vi "Parameter Filter - By Channel Number.vi"(2 "Channel Number":i32, 7 "Parameters Array (in)":T1[](array[typedef])) -> (8 "Filtered Parameters Array (out)":T1[](array[typedef]))   [LabVIEW 2020] (continued)
 "Channel Speed"=100, "Label Decimal"=253, "Label Name"="Label_375", "Min Rate (mS)"=80, "Max Rate (mS)"=120, "SDI"=2, "SSM"=3, "Create SDI"=FALSE, "Create SSM"=FALSE, "Create Parity"=FALSE, "Parameter Name"="eng_rb2_lbl375_b16_28", "Start Bit"=16, "Number of Bits"=13, "Scale"="0.03125", "Offset"="0", "Signed"=TRUE, "Unit"="% Deployed", "Encoding"=enum."BNR", "Default Value"="0"}, {"Core Number"=0, "Channel Number"=23, "Channel Name"="ENG_RB2", "Channel Speed"=100, "Label Decimal"=75, "Label Name"="Label_113", "Min Rate (mS)"=160, "Max Rate (mS)"=240, "SDI"=2, "SSM"=3, "Create SDI"=FALSE, "Create SSM"=FALSE, "Create Parity"=FALSE, "Parameter Name"="eng_rb2_lbl113_b14_27", "Start Bit"=14, "Number of Bits"=14, "Scale"="0.0009765625", "Offset"="0", "Signed"=FALSE, "Unit"="IPS", "Encoding"=enum."BNR", "Default Value"="0"}, {"Core Number"=0, "Channel Number"=23, "Channel Name"="ENG_RB2", "Channel Speed"=100, "Label Decimal"=78, "Label Name"="Label_116", "Min Rate (mS)"=160, "Max Rate (mS)"=240, "SDI"=2, "SSM"=3, "Create SDI"=FALSE, "Create SSM"=FALSE, "Create Parity"=FALSE, "Parameter Name"="eng_rb2_lbl116_b14_27", "Start Bit"=14, "Number of Bits"=14, "Scale"="0.0009765625", "Offset"="0", "Signed"=FALSE, "Unit"="IPS", "Encoding"=enum."BNR", "Default Value"="0"}, {"Core Number"=0, "Channel Number"=23, "Channel Name"="ENG_RB2", "Channel Speed"=100, "Label Decimal"=79, "Label Name"="Label_117", "Min Rate (mS)"=160, "Max Rate (mS)"=240, "SDI"=2, "SSM"=3, "Create SDI"=FALSE, "Create SSM"=FALSE, "Create Parity"=FALSE, "Parameter Name"="eng_rb2_lbl117_b14_27", "Start Bit"=14, "Number of Bits"=14, "Scale"="0.0009765625", "Offset"="0", "Signed"=FALSE, "Unit"="IPS", "Encoding"=enum."BNR", "Default Value"="0"}, {"Core Number"=0, "Channel Number"=23, "Channel Name"="ENG_RB2", "Channel Speed"=100, "Label Decimal"=80, "Label Name"="Label_120", "Min Rate (mS)"=160, "Max Rate (mS)"=240, "SDI"=2, "SSM"=3, "Create SDI"=FALSE, "Create SSM"=FALSE, "Create Parity"=FALSE, "Parameter Name"="eng_rb2_lbl120_b14_27", "Start Bit"=14, "Number of Bits"=14, "Scale"="0.0009765625", "Offset"="0", "Signed"=FALSE, "Unit"="IPS", "Encoding"=enum."BNR", "Default Value"="0"}, {"Core Number"=0, "Channel Number"=23, "Channel Name"="ENG_RB2", "Channel Speed"=100, "Label Decimal"=81, "Label Name"="Label_121", "Min Rate (mS)"=160, "Max Rate (mS)"=240, "SDI"=2, "SSM"=3, "Create SDI"=FALSE, "Create SSM"=FALSE, "Create Parity"=FALSE, "Parameter Name"="eng_rb2_lbl121_b14_27", "Start Bit"=14, "Number of Bits"=14, "Scale"="0.0009765625", "Offset"="0", "Signed"=FALSE, "Unit"="IPS", "Encoding"=enum."BNR", "Default Value"="0"}, {"Core Number"=0, "Channel Number"=23, "Channel Name"="ENG_RB2", "Channel Speed"=100, "Label Decimal"=82, "Label Name"="Label_122", "Min Rate (mS)"=160, "Max Rate (mS)"=240, "SDI"=2, "SSM"=3, "Create SDI"=FALSE, "Create SSM"=FALSE, "Create Parity"=FALSE, "Parameter Name"="eng_rb2_lbl122_b14_27", "Start Bit"=14, "Number of Bits"=14, "Scale"="0.0009765625", "Offset"="0", "Signed"=FALSE, "Unit"="IPS", "Encoding"=enum."BNR", "Default Value"="0"}, {"Core Number"=0, "Channel Number"=23, "Channel Name"="ENG_RB2", "Channel Speed"=100, "Label Decimal"=83, "Label Name"="Label_123", "Min Rate (mS)"=160, "Max Rate (mS)"=240, "SDI"=2, "SSM"=3, "Create SDI"=FALSE, "Create SSM"=FALSE, "Create Parity"=FALSE, "Parameter Name"="eng_rb2_lbl123_b13_27", "Start Bit"=13, "Number of Bits"=15, "Scale"="0.0078125", "Offset"="0", "Signed"=FALSE, "Unit"="% Shaftspeed", "Encoding"=enum."BNR", "Default Value"="0"}, {"Core Number"=0, "Channel Number"=23, "Channel Name"="ENG_RB2", "Channel Speed"=100, "Label Decimal"=84, "Label Name"="Label_124", "Min Rate (mS)"=160, "Max Rate (mS)"=240, "SDI"=2, "SSM"=3, "Create SDI"=FALSE, "Create SSM"=FALSE, "Create Parity"=FALSE, "Parameter Name"="eng_rb2_lbl124_b13_27", "Start Bit"=13, "Number of Bits"=15, "Scale"="0.0078125", "Offset"="0", "Signed"=FALSE, "Unit"="% Shaftspeed", "Encoding"=enum."BNR", "Default Value"="0"}, {"Core Number"=0, "Channel Number"=23, "Channel Name"="ENG_RB2", "Channel Speed"=100, "Label Decimal"=87, "Label Name"="Label_127", "Min Rate (mS)"=160, "Max Rate (mS)"=240, "SDI"=2, "SSM"=3, "Create SDI"=FALSE, "Create SSM"=FALSE, "Create Parity"=FALSE, "Parameter Name"="eng_rb2_lbl127_b19_27", "Start Bit"=19, "Number of Bits"=9, "Scale"="1", "Offset"="0", "Signed"=FALSE, "Unit"="Deg", "Encoding"=enum."BNR", "Default Value"="0"}, {"Core Number"=0, "Channel Number"=23, "Channel Name"="ENG_RB2", "Channel Speed"=100, "Label Decimal"=93, "Label Name"="Label_135", "Min Rate (mS)"=160, "Max Rate (mS)"=240, "SDI"=2, "SSM"=3, "Create SDI"=FALSE, "Create SSM"=FALSE, "Create Parity"=FALSE, "Parameter Name"="eng_rb2_lbl135_b19_27", "Start Bit"=19, "Number of Bits"=9, "Scale"="1", "Offset"="0", "Signed"=FALSE, "Unit"="Deg", "Encoding"=enum."BNR", "Default Value"="0"}, {"Core Number"=0, "Channel Number"=23, "Channel Name"="ENG_RB2", "Channel Speed"=100, "Label Decimal"=94, "Label Name"="Label_136", "Min Rate (mS)"=160, "Max Rate (mS)"=240, "SDI"=2, "SSM"=3, "Create SDI"=FALSE, "Create SSM"=FALSE, "Create Parity"=FALSE, "Parameter Name"="eng_rb2_lbl136_b19_27", "Start Bit"=19, "Number of Bits"=9, "Scale"="1", "Offset"="0", "Signed"=FALSE, "Unit"="Deg", "Encoding"=enum."BNR", "Default Value"="0"}, {"Core Number"=0, "Channel Number"=23, "Channel Name"="ENG_RB2", "Channel Speed"=100, "Label Decimal"=95, "Label Name"="Label_137", "Min Rate (mS)"=160, "Max Rate (mS)"=240, "SDI"=2, "SSM"=3, "Create SDI"=FALSE, "Create SSM"=FALSE, "Create Parity"=FALSE, "Parameter Name"="eng_rb2_lbl137_b19_27", "Start Bit"=19, "Number of Bits"=9, "Scale"="1", "Offset"="0", "Signed"=FALSE, "Unit"="Deg", "Encoding"=enum."BNR", "Default Value"="0"}, {"Core Number"=0, "Channel Number"=23, "Channel Name"="ENG_RB2", "Channel Speed"=100, "Label Decimal"=77, "Label Name"="Label_115", "Min Rate (mS)"=160, "Max Rate (mS)"=240, "SDI"=2, "SSM"=3, "Create SDI"=FALSE, "Create SSM"=FALSE, "Create Parity"=FALSE, "Parameter Name"="eng_rb2_lbl115_b17_28", "Start Bit"=17, "Number of Bits"=12, "Scale"="0.25", "Offset"="0", "Signed"=TRUE, "Unit"="Degrees C", "Encoding"=enum."BNR", "Default Value"="0"}, {"Core Number"=0, "Channel Number"=23, "Channel Name"="ENG_RB2", "Channel Speed"=100, "Label Decimal"=164, "Label Name"="Label_244", "Min Rate (mS)"=160, "Max Rate (mS)"=240, "SDI"=2, "SSM"=3, "Create SDI"=FALSE, "Create SSM"=FALSE, "Create Parity"=FALSE, "Parameter Name"="eng_rb2_lbl244_b12_27", "Start Bit"=12, "Number of Bits"=16, "Scale"="0.25", "Offset"="0", "Signed"=FALSE, "Unit"="pph", "Encoding"=enum."BNR", "Default Value"="0"}, {"Core Number"=0, "Channel Number"=23, "Channel Name"="ENG_RB2", "Channel Speed"=100, "Label Decimal"=206, "Label Name"="Label_316", "Min Rate (mS)"=160, "Max Rate (mS)"=240, "SDI"=2, "SSM"=3, "Create SDI"=FALSE, "Create SSM"=FALSE, "Create Parity"=FALSE, "Parameter Name"="eng_rb2_lbl316_b16_28", "Start Bit"=16, "Number of Bits"=13, "Scale"="0.25", "Offset"="0", "Signed"=TRUE, "Unit"="Degrees C", "Encoding"=enum."BNR", "Default Value"="0"}, {"Core Number"=0, "Channel Number"=23, "Channel Name"="ENG_RB2", "Channel Speed"=100, "Label Decimal"=207, "Label Name"="Label_317", "Min Rate (mS)"=160, "Max Rate (mS)"=240, "SDI"=2, "SSM"=3, "Create SDI"=FALSE, "Create SSM"=FALSE, "Create Parity"=FALSE, "Parameter Name"="eng_rb2_lbl317_b14_27", "Start Bit"=14, "Number of Bits"=14, "Scale"="0.0625", "Offset"="0", "Signed"=FALSE, "Unit"="Psid", "Encoding"=enum."BNR", "Default Value"="0"}, {"Core Number"=0, "Channel Number"=23, "Channel Name"="ENG_RB2", "Channel Speed"=100, "Label Decimal"=162, "Label Name"="Label_242", "Min Rate (mS)"=800, "Max Rate (mS)"=1200, "SDI"=2, "SSM"=3, "Create SDI"=FALSE, "Create SSM"=FALSE, "Create Parity"=FALSE, "Parameter Name"="eng_rb2_lbl242_b18_27", "Start Bit"=18, "Number of Bits"=10, "Scale"="0.0078125", "Offset"="0", "Signed"=FALSE, "Unit"="lbm/s", "Encoding"=enum."BNR", "Default Value"="0"}, {"Core Number"=0, "Channel Number"=23, "Channel Name"="ENG_RB2", "Channel Speed"=100, "Label Decimal"=192, "Label Name"="Label_300", "Min Rate (mS)"=800, "Max Rate (mS)"=1200, "SDI"=2, "SSM"=3, "Create SDI"=FALSE, "Create SSM"=FALSE, "Create Parity"=FALSE, "Parameter Name"="eng_rb2_lbl300_b17_28", "Start Bit"=17, "Number of Bits"=12, "Scale"="0.125", "Offset"="0", "Signed"=TRUE, "Unit"="Deg C", "Encoding"=enum."BNR", "Default Value"="0"}, {"Core Number"=0, "Channel Number"=23, "Channel Name"="ENG_RB2", "Channel Speed"=100, "Label Decimal"=148, "Label Name"="Label_224", "Min Rate (mS)"=800, "Max Rate (mS)"=1200, "SDI"=2, "SSM"=3, "Create SDI"=FALSE, "Create SSM"=FALSE, "Create Parity"=FALSE, "Parameter Name"="eng_rb2_lbl224_b12_27", "Start Bit"=12, "Number of Bits"=16, "Scale"="1", "Offset"="0", "Signed"=FALSE, "Unit"="N/A", "Encoding"=enum."BNR", "Default Value"="0"}, {"Core Number"=0, "Channel Number"=23, "Channel Name"="ENG_RB2", "Channel Speed"=100, "Label Decimal"=149, "Label Name"="Label_225", "Min Rate (mS)"=800, "Max Rate (mS)"=1200, "SDI"=2, "SSM"=3, "Create SDI"=FALSE, "Create SSM"=FALSE, "Create Parity"=FALSE, "Parameter Name"="eng_rb2_lbl225_b12_27", "Start Bit"=12, "Number of Bits"=16, "Scale"="1", "Offset"="0", "Signed"=FALSE, "Unit"="N/A", "Encoding"=enum."BNR", "Default Value"="0"}, {"Core Number"=0, "Channel Number"=23, "Channel Name"="ENG_RB2", "Channel Speed"=100, "Label Decimal"=133, "Label Name"="Label_205", "Min Rate (mS)"=800, "Max Rate (mS)"=1200, "SDI"=2, "SSM"=3, "Create SDI"=FALSE, "Create SSM"=FALSE, "Create Parity"=FALSE, "Parameter Name"="eng_rb2_lbl205_b12_27", "Start Bit"=12, "Number of Bits"=16, "Scale"="0.0000625", "Offset"="0", "Signed"=FALSE, "Unit"="Mach", "Encoding"=enum."BNR", "Default Value"="0"}, {"Core Number"=0, "Channel Number"=23, "Channel Name"="ENG_RB2", "Channel Speed"=100, "Label Decimal"=168, "Label Name"="Label_250", "Min Rate (mS)"=800, "Max Rate (mS)"=1200, "SDI"=2, "SSM"=3, "Create SDI"=FALSE, "Create SSM"=FALSE, "Create Parity"=FALSE, "Parameter Name"="eng_rb2_lbl250_b15_27", "Start Bit"=15, "Number of Bits"=13, "Scale"="0.00048828125", "Offset"="0", "Signed"=FALSE, "Unit"="Pressure ratio", "Encoding"=enum."BNR", "Default Value"="0"}, {"Core Number"=0, "Channel Number"=23, "Channel Name"="ENG_RB2", "Channel Speed"=100, "Label Decimal"=171, "Label Name"="Label_253", "Min Rate (mS)"=800, "Max Rate (mS)"=1200, "SDI"=2, "SSM"=3, "Create SDI"=FALSE, "Create SSM"=FALSE, "Create Parity"=FALSE, "Parameter Name"="eng_rb2_lbl253_b15_27", "Start Bit"=15, "Number of Bits"=13, "Scale"="0.00048828125", "Offset"="0", "Signed"=FALSE, "Unit"="Pressure ratio", "Encoding"=enum."BNR", "Default Value"="0"}, {"Core Number"=0, "Channel Number"=23, "Channel Name"="ENG_RB2", "Channel Speed"=100, "Label Decimal"=173, "Label Name"="Label_255", "Min Rate (mS)"=800, "Max Rate (mS)"=1200, "SDI"=2, "SSM"=3, "Create SDI"=FALSE, "Create SSM"=FALSE, "Create Parity"=FALSE, "Parameter Name"="eng_rb2_lbl255_b15_27", "Start Bit"=15, "Number of Bits"=13, "Scale"="0.00048828125", "Offset"="0", "Signed"=FALSE, "Unit"="Pressure ratio", "Encoding"=enum."BNR", "Default Value"="0"}, {"Core Number"=0, "Channel Number"=23, "Channel Name"="ENG_RB2", "Channel Speed"=100, "Label Decimal"=223, "Label Name"="Label_337", "Min Rate (mS)"=800, "Max Rate (mS)"=1200, "SDI"=2, "SSM"=3, "Create SDI"=FALSE, "Create SSM"=FALSE, "Create Parity"=FALSE, "Parameter Name"="eng_rb2_lbl337_b15_27", "Start Bit"=15, "Number of Bits"=13, "Scale"="0.00048828125", "Offset"="0", "Signed"=FALSE, "Unit"="Pressure ratio", "Encoding"=enum."BNR", "Default Value"="0"}, {"Core Number"=0, "Channel Number"=23, "Channel Name"="ENG_RB2", "Channel Speed"=100, "Label Decimal"=134, "Label Name"="Label_206", "Min Rate (mS)"=800, "Max Rate (mS)"=1200, "SDI"=2, "SSM"=3, "Create SDI"=FALSE, "Create SSM"=FALSE, "Create Parity"=FALSE, "Parameter Name"="eng_rb2_lbl206_b14_27", "Start Bit"=14, "Number of Bits"=14, "Scale"="0.0009765625", "Offset"="0", "Signed"=FALSE, "Unit"="IPS", "Encoding"=enum."BNR", "Default Value"="0"}, {"Core Number"=0, "Channel Number"=23, "Channel Name"="ENG_RB2", "Channel Speed"=100, "Label Decimal"=138, "Label Name"="Label_212", "Min Rate (mS)"=800, "Max Rate (mS)"=1200, "SDI"=2, "SSM"=3, "Create SDI"=FALSE, "Create SSM"=FALSE, "Create Parity"=FALSE, "Parameter Name"="eng_rb2_lbl212_b14_27", "Start Bit"=14, "Number of Bits"=14, "Scale"="0.0009765625", "Offset"="0", "Signed"=FALSE, "Unit"="IPS", "Encoding"=enum."BNR", "Default Value"="0"}, {"Core Number"=0, "Channel Number"=23, "Channel Name"="ENG_RB2", "Channel Speed"=100, "Label Decimal"=65, "Label Name"="Label_101", "Min Rate (mS)"=800, "Max Rate (mS)"=1200, "SDI"=2, "SSM"=3, "Create SDI"=FALSE, "Create SSM"=FALSE, "Create Parity"=FALSE, "Parameter Name"="eng_rb2_lbl101_b12_27", "Start Bit"=12, "Number of Bits"=16, "Scale"="1", "Offset"="0", "Signed"=FALSE, "Unit"="N/A", "Encoding"=enum."BNR", "Default Value"="0"}, {"Core Number"=0, "Channel Number"=23, "Channel Name"="ENG_RB2", "Channel Speed"=100, "Label Decimal"=67, "Label Name"="Label_103", "Min Rate (mS)"=800, "Max Rate (mS)"=1200, "SDI"=2, "SSM"=3, "Create SDI"=FALSE, "Create SSM"=FALSE, "Create Parity"=FALSE, "Parameter Name"="eng_rb2_lbl103_b12_27", "Start Bit"=12, "Number of Bits"=16, "Scale"="1", "Offset"="0", "Signed"=FALSE, "Unit"="N/A", "Encoding"=enum."BNR", "Default Value"="0"}, {"Core Number"=0, "Channel Number"=23, "Channel Name"="ENG_RB2", "Channel Speed"=100, "Label Decimal"=159, "Label Name"="Label_237", "Min Rate (mS)"=800, "Max Rate (mS)"=1200, "SDI"=2, "SSM"=3, "Create SDI"=FALSE, "Create SSM"=FALSE, "Create Parity"=FALSE, "Parameter Name"="eng_rb2_lbl237_b12_27", "Start Bit"=12, "Number of Bits"=16, "Scale"="1", "Offset"="0", "Signed"=FALSE, "Unit"="N/A", "Encoding"=enum."BNR", "Default Value"="0"}, {"Core Number"=0, "Channel Number"=23, "Channel Name"="ENG_RB2", "Channel Speed"=100, "Label Decimal"=214, "Label Name"="Label_326", "Min Rate (mS)"=800, "Max Rate (mS)"=1200, "SDI"=2, "SSM"=3, "Create SDI"=FALSE, "Create SSM"=FALSE, "Create Parity"=FALSE, "Parameter Name"="eng_rb2_lbl326_b12_27", "Start Bit"=12, "Number of Bits"=16, "Scale"="1", "Offset"="0", "Signed"=FALSE, "Unit"="N/A", "Encoding"=enum."BNR", "Default Value"="0"}, {"Core Number"=0, "Channel Number"=23, "Channel Name"="ENG_RB2", "Channel Speed"=100, "Label Decimal"=152, "Label Name"="Label_230", "Min Rate (mS)"=800, "Max Rate (mS)"=1200, "SDI"=2, "SSM"=3, "Create SDI"=FALSE, "Create SSM"=FALSE, "Create Parity"=FALSE, "Parameter Name"="eng_rb2_lbl230_b12_27", "Start Bit"=12, "Number of Bits"=16, "Scale"="1", "Offset"="0", "Signed"=FALSE, "Unit"="N/A", "Encoding"=enum."BNR", "Default Value"="0"}, {"Core Number"=0, "Channel Number"=23, "Channel Name"="ENG_RB2", "Channel Speed"=100, "Label Decimal"=215, "Label Name"="Label_327", "Min Rate (mS)"=800, "Max Rate (mS)"=1200, "SDI"=2, "SSM"=3, "Create SDI"=FALSE, "Create SSM"=FALSE, "Create Parity"=FALSE, "Parameter Name"="eng_rb2_lbl327_b12_27", "Start Bit"=12, "Number of Bits"=16, "Scale"="1", "Offset"="0", "Signed"=FALSE, "Unit"="N/A", "Encoding"=enum."BNR", "Default Value"="0"}, {"Core Number"=0, "Channel Number"=23, "Channel Name"="ENG_RB2", "Channel Speed"=100, "Label Decimal"=154, "Label Name"="Label_232", "Min Rate (mS)"=800, "Max Rate (mS)"=1200, "SDI"=2, "SSM"=3, "Create SDI"=FALSE, "Create SSM"=FALSE, "Create Parity"=FALSE, "Parameter Name"="eng_rb2_lbl232_b12_27", "Start Bit"=12, "Number of Bits"=16, "Scale"="1", "Offset"="0", "Signed"=FALSE, "Unit"="N/A", "Encoding"=enum."BNR", "Default Value"="0"}, {"Core Number"=0, "Channel Number"=23, "Channel Name"="ENG_RB2", "Channel Speed"=100, "Label Decimal"=106, "Label Name"="Label_152", "Min Rate (mS)"=800, "Max Rate (mS)"=1200, "SDI"=2, "SSM"=3, "Create SDI"=FALSE, "Create SSM"=FALSE, "Create Parity"=FALSE, "Parameter Name"="eng_rb2_lbl152_b12_27", "Start Bit"=12, "Number of Bits"=16, "Scale"="1", "Offset"="0", "Signed"=FALSE, "Unit"="N/A", "Encoding"=enum."BNR", "Default Value"="0"}, {"Core Number"=0, "Channel Number"=23, "Channel Name"="ENG_RB2", "Channel Speed"=100, "Label Decimal"=156, "Label Name"="Label_234", "Min Rate (mS)"=800, "Max Rate (mS)"=1200, "SDI"=2, "SSM"=3, "Create SDI"=FALSE, "Create SSM"=FALSE, "Create Parity"=FALSE, "Parameter Name"="eng_rb2_lbl234_b12_27", "Start Bit"=12, "Number of Bits"=16, "Scale"="1", "Offset"="0", "Signed"=FALSE, "Unit"="N/A", "Encoding"=enum."BNR", "Default Value"="0"}, {"Core Number"=0, "Channel Number"=23, "Channel Name"="ENG_RB2", "Channel Speed"=100, "Label Decimal"=135, "Label Name"="Label_207", "Min Rate (mS)"=800, "Max Rate (mS)"=1200, "SDI"=2, "SSM"=3, "Create SDI"=FALSE, "Create SSM"=FALSE, "Create Parity"=FALSE, "Parameter Name"="eng_rb2_lbl207_b12_27", "Start Bit"=12, "Number of Bits"=16, "Scale"="1", "Offset"="0", "Signed"=FALSE, "Unit"="N/A", "Encoding"=enum."BNR", "Default Value"="0"}, {"Core Number"=0, "Channel Number"=23, "Channel Name"="ENG_RB2", "Channel Speed"=100, "Label Decimal"=157, "Label Name"="Label_235", "Min Rate (mS)"=800, "Max Rate (mS)"=1200, "SDI"=2, "SSM"=3, "Create SDI"=FALSE, "Create SSM"=FALSE, "Create Parity"=FALSE, "Parameter Name"="eng_rb2_lbl235_b14_28", "Start Bit"=14, "Number of Bits"=15, "Scale"="0.0067138671875", "Offset"="0", "Signed"=TRUE, "Unit"="Psia", "Encoding"=enum."BNR", "Default Value"="0"}, {"Core Number"=0, "Channel Number"=23, "Channel Name"="ENG_RB2", "Channel Speed"=100, "Label Decimal"=43, "Label Name"="Label_53", "Min Rate (mS)"=800, "Max Rate (mS)"=1200, "SDI"=2, "SSM"=3, "Create SDI"=FALSE, "Create SSM"=FALSE, "Create Parity"=FALSE, "Parameter Name"="eng_rb2_lbl53_b14_27", "Start Bit"=14, "Number of Bits"=14, "Scale"="0.001953125", "Offset"="0", "Signed"=FALSE, "Unit"="Psia", "Encoding"=enum."BNR", "Default Value"="0"}, {"Core Number"=0, "Channel Number"=23, "Channel Name"="ENG_RB2", "Channel Speed"=100, "Label Decimal"=76, "Label Name"="Label_114", "Min Rate (mS)"=800, "Max Rate (mS)"=1200, "SDI"=2, "SSM"=3, "Create SDI"=FALSE, "Create SSM"=FALSE, "Create Parity"=FALSE, "Parameter Name"="eng_rb2_lbl114_b14_27", "Start Bit"=14, "Number of Bits"=14, "Scale"="0.001953125", "Offset"="0", "Signed"=FALSE, "Unit"="Psia", "Encoding"=enum."BNR", "Default Value"="0"}, {"Core Number"=0, "Channel Number"=23, "Channel Name"="ENG_RB2", "Channel Speed"=100, "Label Decimal"=131, "Label Name"="Label_203", "Min Rate (mS)"=800, "Max Rate (mS)"=1200, "SDI"=2, "SSM"=3, "Create SDI"=FALSE, "Create SSM"=FALSE, "Create Parity"=FALSE, "Parameter Name"="eng_rb2_lbl203_b13_28", "Start Bit"=13, "Number of Bits"=16, "Scale"="2", "Offset"="0", "Signed"=TRUE, "Unit"="Feet", "Encoding"=enum."BNR", "Default Value"="0"}, {"Core Number"=0, "Channel Number"=23, "Channel Name"="ENG_RB2", "Channel Speed"=100, "Label Decimal"=153, "Label Name"="Label_231", "Min Rate (mS)"=800, "Max Rate (mS)"=1200, "SDI"=2, "SSM"=3, "Create SDI"=FALSE, "Create SSM"=FALSE, "Create Parity"=FALSE, "Parameter Name"="eng_rb2_lbl231_b17_28", "Start Bit"=17, "Number of Bits"=12, "Scale"="0.125", "Offset"="0", "Signed"=TRUE, "Unit"="Degrees C", "Encoding"=enum."BNR", "Default Value"="0"}, {"Core Number"=0, "Channel Number"=23, "Channel Name"="ENG_RB2", "Channel Speed"=100, "Label Decimal"=195, "Label Name"="Label_303", "Min Rate (mS)"=800, "Max Rate (mS)"=1200, "SDI"=2, "SSM"=3, "Create SDI"=FALSE, "Create SSM"=FALSE, "Create Parity"=FALSE, "Parameter Name"="eng_rb2_lbl303_b15_27", "Start Bit"=15, "Number of Bits"=13, "Scale"="0.00390625", "Offset"="0", "Signed"=FALSE, "Unit"="Psia", "Encoding"=enum."BNR", "Default Value"="0"}, {"Core Number"=0, "Channel Number"=23, "Channel Name"="ENG_RB2", "Channel Speed"=100, "Label Decimal"=24, "Label Name"="Label_30", "Min Rate (mS)"=800, "Max Rate (mS)"=1200, "SDI"=2, "SSM"=3, "Create SDI"=FALSE, "Create SSM"=FALSE, "Create Parity"=FALSE, "Parameter Name"="eng_rb2_lbl30_b14_27", "Start Bit"=14, "Number of Bits"=14, "Scale"="0.03125", "Offset"="0", "Signed"=FALSE, "Unit"="Psid", "Encoding"=enum."BNR", "Default Value"="0"}, {"Core Number"=0, "Channel Number"=23, "Channel Name"="ENG_RB2", "Channel Speed"=100, "Label Decimal"=40, "Label Name"="Label_50", "Min Rate (mS)"=800, "Max Rate (mS)"=1200, "SDI"=2, "SSM"=3, "Create SDI"=FALSE, "Create SSM"=FALSE, "Create Parity"=FALSE, "Parameter Name"="eng_rb2_lbl50_b14_27", "Start Bit"=14, "Number of Bits"=14, "Scale"="0.015625", "Offset"="0", "Signed"=FALSE, "Unit"="% Shaftspeed", "Encoding"=enum."BNR", "Default Value"="0"}, {"Core Number"=0, "Channel Number"=23, "Channel Name"="ENG_RB2", "Channel Speed"=100, "Label Decimal"=41, "Label Name"="Label_51", "Min Rate (mS)"=800, "Max Rate (mS)"=1200, "SDI"=2, "SSM"=3, "Create SDI"=FALSE, "Create SSM"=FALSE, "Create Parity"=FALSE, "Parameter Name"="eng_rb2_lbl51_b14_27", "Start Bit"=14, "Number of Bits"=14, "Scale"="0.015625", "Offset"="0", "Signed"=FALSE, "Unit"="% Shaftspeed", "Encoding"=enum."BNR", "Default Value"="0"}, {"Core Number"=0, "Channel Number"=23, "Channel Name"="ENG_RB2", "Channel Speed"=100, "Label Decimal"=85, "Label Name"="Label_125", "Min Rate (mS)"=800, "Max Rate (mS)"=1200, "SDI"=2, "SSM"=3, "Create SDI"=FALSE, "Create SSM"=FALSE, "Create Parity"=FALSE, "Parameter Name"="eng_rb2_lbl125_b16_28", "Start Bit"=16, "Number of Bits"=13, "Scale"="0.125", "Offset"="0", "Signed"=TRUE, "Unit"="Degrees C", "Encoding"=enum."BNR", "Default Value"="0"}, {"Core Number"=0, "Channel Number"=23, "Channel Name"="ENG_RB2", "Channel Speed"=100, "Label Decimal"=86, "Label Name"="Label_126", "Min Rate (mS)"=800, "Max Rate (mS)"=1200, "SDI"=2, "SSM"=3, "Create SDI"=FALSE, "Create SSM"=FALSE, "Create Parity"=FALSE, "Parameter Name"="eng_rb2_lbl126_b16_28", "Start Bit"=16, "Number of Bits"=13, "Scale"="0.125", "Offset"="0", "Signed"=TRUE, "Unit"="Degrees C", "Encoding"=enum."BNR", "Default Value"="0"}, {"Core Number"=0, "Channel Number"=23, "Channel Name"="ENG_RB2", "Channel Speed"=100, "Label Decimal"=96, "Label Name"="Label_140", "Min Rate (mS)"=800, "Max Rate (mS)"=1200, "SDI"=2, "SSM"=3, "Create SDI"=FALSE, "Create SSM"=FALSE, "Create Parity"=FALSE, "Parameter Name"="eng_rb2_lbl140_b15_28", "Start Bit"=15, "Number of Bits"=14, "Scale"="0.5", "Offset"="0", "Signed"=TRUE, "Unit"="Degrees C", "Encoding"=enum."BNR", "Default Value"="0"}, {"Core Number"=0, "Channel Number"=23, "Channel Name"="ENG_RB2", "Channel Speed"=100, "Label Decimal"=116, "Label Name"="Label_164", "Min Rate (mS)"=800, "Max Rate (mS)"=1200, "SDI"=2, "SSM"=3, "Create SDI"=FALSE, "Create SSM"=FALSE, "Create Parity"=FALSE, "Parameter Name"="eng_rb2_lbl164_b14_27", "Start Bit"=14, "Number of Bits"=14, "Scale"="0.03125", "Offset"="0", "Signed"=FALSE, "Unit"="Psid", "Encoding"=enum."BNR", "Default Value"="0"}, {"Core Number"=0, "Channel Number"=23, "Channel Name"="ENG_RB2", "Channel Speed"=100, "Label Decimal"=121, "Label Name"="Label_171", "Min Rate (mS)"=800, "Max Rate (mS)"=1200, "SDI"=2, "SSM"=3, "Create SDI"=FALSE, "Create SSM"=FALSE, "Create Parity"=FALSE, "Parameter Name"="eng_rb2_lbl171_b14_27", "Start Bit"=14, "Number of Bits"=14, "Scale"="0.015625", "Offset"="0", "Signed"=FALSE, "Unit"="% Shaftspeed", "Encoding"=enum."BNR", "Default Value"="0"}, {"Core Number"=0, "Channel Number"=23, "Channel Name"="ENG_RB2", "Channel Speed"=100, "Label Decimal"=122, "Label Name"="Label_172", "Min Rate (mS)"=800, "Max Rate (mS)"=1200, "SDI"=2, "SSM"=3, "Create SDI"=FALSE, "Create SSM"=FALSE, "Create Parity"=FALSE, "Parameter Name"="eng_rb2_lbl172_b14_27", "Start Bit"=14, "Number of Bits"=14, "Scale"="0.015625", "Offset"="0", "Signed"=FALSE, "Unit"="% Shaftspeed", "Encoding"=enum."BNR", "Default Value"="0"}, {"Core Number"=0, "Channel Number"=23, "Channel Name"="ENG_RB2", "Channel Speed"=100, "Label Decimal"=123, "Label Name"="Label_173", "Min Rate (mS)"=800, "Max Rate (mS)"=1200, "SDI"=2, "SSM"=3, "Create SDI"=FALSE, "Create SSM"=FALSE, "Create Parity"=FALSE, "Parameter Name"="eng_rb2_lbl173_b14_27", "Start Bit"=14, "Number of Bits"=14, "Scale"="0.015625", "Offset"="0", "Signed"=FALSE, "Unit"="% Shaftspeed", "Encoding"=enum."BNR", "Default Value"="0"}, {"Core Number"=0, "Channel Number"=23, "Channel Name"="ENG_RB2", "Channel Speed"=100, "Label Decimal"=124, "Label Name"="Label_174", "Min Rate (mS)"=800, "Max Rate (mS)"=1200, "SDI"=2, "SSM"=3, "Create SDI"=FALSE, "Create SSM"=FALSE, "Create Parity"=FALSE, "Parameter Name"="eng_rb2_lbl174_b14_27", "Start Bit"=14, "Number of Bits"=14, "Scale"="0.015625", "Offset"="0", "Signed"=FALSE, "Unit"="% Shaftspeed", "Encoding"=enum."BNR", "Default Value"="0"}, {"Core Number"=0, "Channel Number"=23, "Channel Name"="ENG_RB2", "Channel Speed"=100, "Label Decimal"=128, "Label Name"="Label_200", "Min Rate (mS)"=800, "Max Rate (mS)"=1200, "SDI"=2, "SSM"=3, "Create SDI"=FALSE, "Create SSM"=FALSE, "Create Parity"=FALSE, "Parameter Name"="eng_rb2_lbl200_b16_28", "Start Bit"=16, "Number of Bits"=13, "Scale"="0.125", "Offset"="0", "Signed"=TRUE, "Unit"="Degrees C", "Encoding"=enum."BNR", "Default Value"="0"}, {"Core Number"=0, "Channel Number"=23, "Channel Name"="ENG_RB2", "Channel Speed"=100, "Label Decimal"=160, "Label Name"="Label_240", "Min Rate (mS)"=800, "Max Rate (mS)"=1200, "SDI"=2, "SSM"=3, "Create SDI"=FALSE, "Create SSM"=FALSE, "Create Parity"=FALSE, "Parameter Name"="eng_rb2_lbl240_b15_28", "Start Bit"=15, "Number of Bits"=14, "Scale"="0.5", "Offset"="0", "Signed"=TRUE, "Unit"="Degrees C", "Encoding"=enum."BNR", "Default Value"="0"}, {"Core Number"=0, "Channel Number"=23, "Channel Name"="ENG_RB2", "Channel Speed"=100, "Label Decimal"=163, "Label Name"="Label_243", "Min Rate (mS)"=800, "Max Rate (mS)"=1200, "SDI"=2, "SSM"=3, "Create SDI"=FALSE, "Create SSM"=FALSE, "Create Parity"=FALSE, "Parameter Name"="eng_rb2_lbl243_b15_28", "Start Bit"=15, "Number of Bits"=14, "Scale"="0.5", "Offset"="0", "Signed"=TRUE, "Unit"="Degrees C", "Encoding"=enum."BNR", "Default Value"="0"}, {"Core Number"=0, "Channel Number"=23, "Channel Name"="ENG_RB2", "Channel Speed"=100, "Label Decimal"=72, "Label Name"="Label_110", "Min Rate (mS)"=800, "Max Rate (mS)"=1200, "SDI"=2, "SSM"=3, "Create SDI"=FALSE, "Create SSM"=FALSE, "Create Parity"=FALSE, "Parameter Name"="eng_rb2_lbl110_b20_28", "Start Bit"=20, "Number of Bits"=9, "Scale"="2", "Offset"="0", "Signed"=TRUE, "Unit"="Psig", "Encoding"=enum."BNR", "Default Value"="0"}, {"Core Number"=0, "Channel Number"=23, "Channel Name"="ENG_RB2", "Channel Speed"=100, "Label Decimal"=89, "Label Name"="Label_131", "Min Rate (mS)"=800, "Max Rate (mS)"=1200, "SDI"=2, "SSM"=3, "Create SDI"=FALSE, "Create SSM"=FALSE, "Create Parity"=FALSE, "Parameter Name"="eng_rb2_lbl131_b15_27", "Start Bit"=15, "Number of Bits"=13, "Scale"="0.015625", "Offset"="0", "Signed"=FALSE, "Unit"="Psid", "Encoding"=enum."BNR", "Default Value"="0"}, {"Core Number"=0, "Channel Number"=23, "Channel Name"="ENG_RB2", "Channel Speed"=100, "Label Decimal"=137, "Label Name"="Label_211", "Min Rate (mS)"=800, "Max Rate (mS)"=1200, "SDI"=2, "SSM"=3, "Create SDI"=FALSE, "Create SSM"=FALSE, "Create Parity"=FALSE, "Parameter Name"="eng_rb2_lbl211_b20_28", "Start Bit"=20, "Number of Bits"=9, "Scale"="0.25", "Offset"="0", "Signed"=TRUE, "Unit"="Psid", "Encoding"=enum."BNR", "Default Value"="0"}, {"Core Number"=0, "Channel Number"=23, "Channel Name"="ENG_RB2", "Channel Speed"=100, "Label Decimal"=92, "Label Name"="Label_134", "Min Rate (mS)"=800, "Max Rate (mS)"=1200, "SDI"=2, "SSM"=3, "Create SDI"=FALSE, "Create SSM"=FALSE, "Create Parity"=FALSE, "Parameter Name"="eng_rb2_lbl134_b13_28", "Start Bit"=13, "Number of Bits"=16, "Scale"="0.03125", "Offset"="0", "Signed"=TRUE, "Unit"="Degrees", "Encoding"=enum."BNR", "Default Value"="0"}, {"Core Number"=0, "Channel Number"=23, "Channel Name"="ENG_RB2", "Channel Speed"=100, "Label Decimal"=60, "Label Name"="Label_74", "Min Rate (mS)"=800, "Max Rate (mS)"=1200, "SDI"=2, "SSM"=3, "Create SDI"=FALSE, "Create SSM"=FALSE, "Create Parity"=FALSE, "Parameter Name"="eng_rb2_lbl74_b15_28", "Start Bit"=15, "Number of Bits"=14, "Scale"="0.00390625", "Offset"="0", "Signed"=TRUE, "Unit"="US pints below full", "Encoding"=enum."BNR", "Default Value"="0"}, {"Core Number"=0, "Channel Number"=23, "Channel Name"="ENG_RB2", "Channel Speed"=100, "Label Decimal"=196, "Label Name"="Label_304", "Min Rate (mS)"=800, "Max Rate (mS)"=1200, "SDI"=2, "SSM"=3, "Create SDI"=FALSE, "Create SSM"=FALSE, "Create Parity"=FALSE, "Parameter Name"="eng_rb2_lbl304_b14_28", "Start Bit"=14, "Number of Bits"=15, "Scale"="0.0078125", "Offset"="0", "Signed"=TRUE, "Unit"="Psid", "Encoding"=enum."BNR", "Default Value"="0"}, {"Core Number"=0, "Channel Number"=23, "Channel Name"="ENG_RB2", "Channel Speed"=100, "Label Decimal"=170, "Label Name"="Label_252", "Min Rate (mS)"=800, "Max Rate (mS)"=1200, "SDI"=2, "SSM"=3, "Create SDI"=FALSE, "Create SSM"=FALSE, "Create Parity"=FALSE, "Parameter Name"="eng_rb2_lbl252_b16_27", "Start Bit"=16, "Number of Bits"=12, "Scale"="0.0009765625", "Offset"="0", "Signed"=FALSE, "Unit"="Pressure ratio", "Encoding"=enum."BNR", "Default Value"="0"}, {"Core Number"=0, "Channel Number"=23, "Channel Name"="ENG_RB2", "Channel Speed"=100, "Label Decimal"=48, "Label Name"="Label_60", "Min Rate (mS)"=800, "Max Rate (mS)"=1200, "SDI"=2, "SSM"=3, "Create SDI"=FALSE, "Create SSM"=FALSE, "Create Parity"=FALSE, "Parameter Name"="eng_rb2_lbl60_b13_27", "Start Bit"=13, "Number of Bits"=15, "Scale"="1", "Offset"="0", "Signed"=FALSE, "Unit"="N/A", "Encoding"=enum."BNR", "Default Value"="0"}, {"Core Number"=0, "Channel Number"=23, "Channel Name"="ENG_RB2", "Channel Speed"=100, "Label Decimal"=150, "Label Name"="Label_226", "Min Rate (mS)"=800, "Max Rate (mS)"=1200, "SDI"=2, "SSM"=3, "Create SDI"=FALSE, "Create SSM"=FALSE, "Create Parity"=FALSE, "Parameter Name"="eng_rb2_lbl226_b13_27", "Start Bit"=13, "Number of Bits"=15, "Scale"="1", "Offset"="0", "Signed"=FALSE, "Unit"="N/A", "Encoding"=enum."BNR", "Default Value"="0"}, {"Core Number"=0, "Channel Number"=23, "Channel Name"="ENG_RB2", "Channel Speed"=100, "Label Decimal"=151, "Label Name"="Label_227", "Min Rate (mS)"=800, "Max Rate (mS)"=1200, "SDI"=2, "SSM"=3, "Create SDI"=FALSE, "Create SSM"=FALSE, "Create Parity"=FALSE, "Parameter Name"="eng_rb2_lbl227_b13_27", "Start Bit"=13, "Number of Bits"=15, "Scale"="1", "Offset"="0", "Signed"=FALSE, "Unit"="N/A", "Encoding"=enum."BNR", "Default Value"="0"}, {"Core Number"=0, "Channel Number"=23, "Channel Name"="ENG_RB2", "Channel Speed"=100, "Label Decimal"=158, "Label Name"="Label_236", "Min Rate (mS)"=800, "Max Rate (mS)"=1200, "SDI"=2, "SSM"=3, "Create SDI"=FALSE, "Create SSM"=FALSE, "Create Parity"=FALSE, "Parameter Name"="eng_rb2_lbl236_b13_27", "Start Bit"=13, "Number of Bits"=15, "Scale"="1", "Offset"="0", "Signed"=FALSE, "Unit"="N/A", "Encoding"=enum."BNR", "Default Value"="0"}, {"Core Number"=0, "Channel Number"=23, "Channel Name"="ENG_RB2", "Channel Speed"=100, "Label Decimal"=184, "Label Name"="Label_270", "Min Rate (mS)"=40, "Max Rate (mS)"=60, "SDI"=2, "SSM"=0, "Create SDI"=FALSE, "Create SSM"=FALSE, "Create Parity"=FALSE, "Parameter Name"="eng_rb2_lbl270_b10_28", "Start Bit"=10, "Number of Bits"=19, "Scale"="1", "Offset"="0", "Signed"=FALSE, "Unit"="N/A", "Encoding"=enum."Discrete", "Default Value"="0"}, {"Core Number"=0, "Channel Number"=23, "Channel Name"="ENG_RB2", "Channel Speed"=100, "Label Decimal"=232, "Label Name"="Label_350", "Min Rate (mS)"=160, "Max Rate (mS)"=240, "SDI"=2, "SSM"=0, "Create SDI"=FALSE, "Create SSM"=FALSE, "Create Parity"=FALSE, "Parameter Name"="eng_rb2_lbl350_b10_28", "Start Bit"=10, "Number of Bits"=19, "Scale"="1", "Offset"="0", "Signed"=FALSE, "Unit"="N/A", "Encoding"=enum."Discrete", "Default Value"="0"}, {"Core Number"=0, "Channel Number"=23, "Channel Name"="ENG_RB2", "Channel Speed"=100, "Label Decimal"=185, "Label Name"="Label_271", "Min Rate (mS)"=160, "Max Rate (mS)"=240, "SDI"=2, "SSM"=0, "Create SDI"=FALSE, "Create SSM"=FALSE, "Create Parity"=FALSE, "Parameter Name"="eng_rb2_lbl271_b10_28", "Start Bit"=10, "Number of Bits"=19, "Scale"="1", "Offset"="0", "Signed"=FALSE, "Unit"="N/A", "Encoding"=enum."Discrete", "Default Value"="0"}, {"Core Number"=0, "Channel Number"=23, "Channel Name"="ENG_RB2", "Channel Speed"=100, "Label Decimal"=186, "Label Name"="Label_272", "Min Rate (mS)"=160, "Max Rate (mS)"=240, "SDI"=2, "SSM"=0, "Create SDI"=FALSE, "Create SSM"=FALSE, "Create Parity"=FALSE, "Parameter Name"="eng_rb2_lbl272_b10_28", "Start Bit"=10, "Number of Bits"=19, "Scale"="1", "Offset"="0", "Signed"=FALSE, "Unit"="N/A", "Encoding"=enum."Discrete", "Default Value"="0"}, {"Core Number"=0, "Channel Number"=23, "Channel Name"="ENG_RB2", "Channel Speed"=100, "Label Decimal"=187, "Label Name"="Label_273", "Min Rate (mS)"=160, "Max Rate (mS)"=240, "SDI"=2, "SSM"=0, "Create SDI"=FALSE, "Create SSM"=FALSE, "Create Parity"=FALSE, "Parameter Name"="eng_rb2_lbl273_b10_28", "Start Bit"=10, "Number of Bits"=19, "Scale"="1", "Offset"="0", "Signed"=FALSE, "Unit"="N/A", "Encoding"=enum."Discrete", "Default Value"="0"}, {"Core Number"=0, "Channel Number"=23, "Channel Name"="ENG_RB2", "Channel Speed"=100, "Label Decimal"=188, "Label Name"="Label_274", "Min Rate (mS)"=160, "Max Rate (mS)"=240, "SDI"=2, "SSM"=0, "Create SDI"=FALSE, "Create SSM"=FALSE, "Create Parity"=FALSE, "Parameter Name"="eng_rb2_lbl274_b10_28", "Start Bit"=10, "Number of Bits"=19, "Scale"="1", "Offset"="0", "Signed"=FALSE, "Unit"="N/A", "Encoding"=enum."Discrete", "Default Value"="0"}, {"Core Number"=0, "Channel Number"=23, "Channel Name"="ENG_RB2", "Channel Speed"=100, "Label Decimal"=189, "Label Name"="Label_275", "Min Rate (mS)"=160, "Max Rate (mS)"=240, "SDI"=2, "SSM"=0, "Create SDI"=FALSE, "Create SSM"=FALSE, "Create Parity"=FALSE, "Parameter Name"="eng_rb2_lbl275_b10_28", "Start Bit"=10, "Number of Bits"=19, "Scale"="1", "Offset"="0", "Signed"=FALSE, "Unit"="N/A", "Encoding"=enum."Discrete", "Default Value"="0"}, {"Core Number"=0, "Channel Number"=23, "Channel Name"="ENG_RB2", "Channel Speed"=100, "Label Decimal"=190, "Label Name"="Label_276", "Min Rate (mS)"=160, "Max Rate (mS)"=240, "SDI"=2, "SSM"=0, "Create SDI"=FALSE, "Create SSM"=FALSE, "Create Parity"=FALSE, "Parameter Name"="eng_rb2_lbl276_b10_28", "Start Bit"=10, "Number of Bits"=19, "Scale"="1", "Offset"="0", "Signed"=FALSE, "Unit"="N/A", "Encoding"=enum."Discrete", "Default Value"="0"}, {"Core Number"=0, "Channel Number"=23, "Channel Name"="ENG_RB2", "Channel Speed"=100, "Label Decimal"=191, "Label Name"="Label_277", "Min Rate (mS)"=160, "Max Rate (mS)"=240, "SDI"=2, "SSM"=0, "Create SDI"=FALSE, "Create SSM"=FALSE, "Create Parity"=FALSE, "Parameter Name"="eng_rb2_lbl277_b10_28", "Start Bit"=10, "Number of Bits"=19, "Scale"="1", "Offset"="0", "Signed"=FALSE, "Unit"="N/A", "Encoding"=enum."Discrete", "Default Value"="0"}, {"Core Number"=0, "Channel Number"=23, "Channel Name"="ENG_RB2", "Channel Speed"=100, "Label Decimal"=254, "Label Name"="Label_376", "Min Rate (mS)"=160, "Max Rate (mS)"=240, "SDI"=2, "SSM"=0, "Create SDI"=FALSE, "Create SSM"=FALSE, "Create Parity"=FALSE, "Parameter Name"="eng_rb2_lbl376_b10_28", "Start Bit"=10, "Number of Bits"=19, "Scale"="1", "Offset"="0", "Signed"=FALSE, "Unit"="N/A", "Encoding"=enum."Discrete", "Default Value"="0"}, {"Core Number"=0, "Channel Number"=23, "Channel Name"="ENG_RB2", "Channel Speed"=100, "Label Decimal"=104, "Label Name"="Label_150", "Min Rate (mS)"=720, "Max Rate (mS)"=1080, "SDI"=2, "SSM"=0, "Create SDI"=FALSE, "Create SSM"=FALSE, "Create Parity"=FALSE, "Parameter Name"="eng_rb2_lbl150_b10_28", "Start Bit"=10, "Number of Bits"=19, "Scale"="1", "Offset"="0", "Signed"=FALSE, "Unit"="N/A", "Encoding"=enum."Discrete", "Default Value"="0"}, {"Core Number"=0, "Channel Number"=23, "Channel Name"="ENG_RB2", "Channel Speed"=100, "Label Decimal"=105, "Label Name"="Label_151", "Min Rate (mS)"=720, "Max Rate (mS)"=1080, "SDI"=2, "SSM"=0, "Create SDI"=FALSE, "Create SSM"=FALSE, "Create Parity"=FALSE, "Parameter Name"="eng_rb2_lbl151_b10_28", "Start Bit"=10, "Number of Bits"=19, "Scale"="1", "Offset"="0", "Signed"=FALSE, "Unit"="N/A", "Encoding"=enum."Discrete", "Default Value"="0"}, {"Core Number"=0, "Channel Number"=23, "Channel Name"="ENG_RB2", "Channel Speed"=100, "Label Decimal"=107, "Label Name"="Label_153", "Min Rate (mS)"=720, "Max Rate (mS)"=1080, "SDI"=2, "SSM"=0, "Create SDI"=FALSE, "Create SSM"=FALSE, "Create Parity"=FALSE, "Parameter Name"="eng_rb2_lbl153_b10_28", "Start Bit"=10, "Number of Bits"=19, "Scale"="1", "Offset"="0", "Signed"=FALSE, "Unit"="N/A", "Encoding"=enum."Discrete", "Default Value"="0"}, {"Core Number"=0, "Channel Number"=23, "Channel Name"="ENG_RB2", "Channel Speed"=100, "Label Decimal"=108, "Label Name"="Label_154", "Min Rate (mS)"=720, "Max Rate (mS)"=1080, "SDI"=2, "SSM"=0, "Create SDI"=FALSE, "Create SSM"=FALSE, "Create Parity"=FALSE, "Parameter Name"="eng_rb2_lbl154_b10_28", "Start Bit"=10, "Number of Bits"=19, "Scale"="1", "Offset"="0", "Signed"=FALSE, "Unit"="N/A", "Encoding"=enum."Discrete", "Default Value"="0"}, {"Core Number"=0, "Channel Number"=23, "Channel Name"="ENG_RB2", "Channel Speed"=100, "Label Decimal"=109, "Label Name"="Label_155", "Min Rate (mS)"=720, "Max Rate (mS)"=1080, "SDI"=2, "SSM"=0, "Create SDI"=FALSE, "Create SSM"=FALSE, "Create Parity"=FALSE, "Parameter Name"="eng_rb2_lbl155_b10_28", "Start Bit"=10, "Number of Bits"=19, "Scale"="1", "Offset"="0", "Signed"=FALSE, "Unit"="N/A", "Encoding"=enum."Discrete", "Default Value"="0"}, {"Core Number"=0, "Channel Number"=23, "Channel Name"="ENG_RB2", "Channel Speed"=100, "Label Decimal"=110, "Label Name"="Label_156", "Min Rate (mS)"=720, "Max Rate (mS)"=1080, "SDI"=2, "SSM"=0, "Create SDI"=FALSE, "Create SSM"=FALSE, "Create Parity"=FALSE, "Parameter Name"="eng_rb2_lbl156_b10_28", "Start Bit"=10, "Number of Bits"=19, "Scale"="1", "Offset"="0", "Signed"=FALSE, "Unit"="N/A", "Encoding"=enum."Discrete", "Default Value"="0"}, {"Core Number"=0, "Channel Number"=23, "Channel Name"="ENG_RB2", "Channel Speed"=100, "Label Decimal"=111, "Label Name"="Label_157", "Min Rate (mS)"=720, "Max Rate (mS)"=1080, "SDI"=2, "SSM"=0, "Create SDI"=FALSE, "Create SSM"=FALSE, "Create Parity"=FALSE, "Parameter Name"="eng_rb2_lbl157_b10_28", "Start Bit"=10, "Number of Bits"=19, "Scale"="1", "Offset"="0", "Signed"=FALSE, "Unit"="N/A", "Encoding"=enum."Discrete", "Default Value"="0"}, {"Core Number"=0, "Channel Number"=23, "Channel Name"="ENG_RB2", "Channel Speed"=100, "Label Decimal"=112, "Label Name"="Label_160", "Min Rate (mS)"=720, "Max Rate (mS)"=1080, "SDI"=2, "SSM"=0, "Create SDI"=FALSE, "Create SSM"=FALSE, "Create Parity"=FALSE, "Parameter Name"="eng_rb2_lbl160_b10_28", "Start Bit"=10, "Number of Bits"=19, "Scale"="1", "Offset"="0", "Signed"=FALSE, "Unit"="N/A", "Encoding"=enum."Discrete", "Default Value"="0"}, {"Core Number"=0, "Channel Number"=23, "Channel Name"="ENG_RB2", "Channel Speed"=100, "Label Decimal"=113, "Label Name"="Label_161", "Min Rate (mS)"=720, "Max Rate (mS)"=1080, "SDI"=2, "SSM"=0, "Create SDI"=FALSE, "Create SSM"=FALSE, "Create Parity"=FALSE, "Parameter Name"="eng_rb2_lbl161_b10_28", "Start Bit"=10, "Number of Bits"=19, "Scale"="1", "Offset"="0", "Signed"=FALSE, "Unit"="N/A", "Encoding"=enum."Discrete", "Default Value"="0"}, {"Core Number"=0, "Channel Number"=23, "Channel Name"="ENG_RB2", "Channel Speed"=100, "Label Decimal"=114, "Label Name"="Label_162", "Min Rate (mS)"=720, "Max Rate (mS)"=1080, "SDI"=2, "SSM"=0, "Create SDI"=FALSE, "Create SSM"=FALSE, "Create Parity"=FALSE, "Parameter Name"="eng_rb2_lbl162_b10_28", "Start Bit"=10, "Number of Bits"=19, "Scale"="1", "Offset"="0", "Signed"=FALSE, "Unit"="N/A", "Encoding"=enum."Discrete", "Default Value"="0"}, {"Core Number"=0, "Channel Number"=23, "Channel Name"="ENG_RB2", "Channel Speed"=100, "Label Decimal"=115, "Label Name"="Label_163", "Min Rate (mS)"=720, "Max Rate (mS)"=1080, "SDI"=2, "SSM"=0, "Create SDI"=FALSE, "Create SSM"=FALSE, "Create Parity"=FALSE, "Parameter Name"="eng_rb2_lbl163_b10_28", "Start Bit"=10, "Number of Bits"=19, "Scale"="1", "Offset"="0", "Signed"=FALSE, "Unit"="N/A", "Encoding"=enum."Discrete", "Default Value"="0"}, {"Core Number"=0, "Channel Number"=23, "Channel Name"="ENG_RB2", 
